vi "Is valid.vi"(11 "address":refnum<class "MacOS Network Address.lvclass">) -> (2 "valid?":bool, 3 "address out":refnum<class "MacOS Network Address.lvclass">)   [LabVIEW 2020, in "NI_WFCN.lvlib" / "MacOS Network Address.lvclass"]
doc: "Does this object actually store a network address? (If FALSE, this object is just a stub.)"
uses:
  <vilib>/net/WFCN/Addressing/MacOS Network Address/MacOS Network Address.lvclass
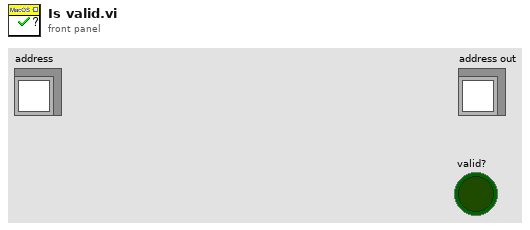
[diagram p1: front panel]
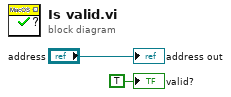
[diagram p0: block diagram]
diagram:
  "address out" <- "address"
  "valid?" <- TRUE ("valid?")
